vi "AuMT8852B Single-slot Sensitivity Results Query.vi"(8 "error in (no error)":errorcluster, 11 "VISA session":refnum<visa-resource-name>) -> (0 "error out":errorcluster, 2 "error code":i32, 3 "VISA session out":refnum<visa-resource-name>, 4 "Results":T1 {"Overall FER" format="%.2f"; "Current FER" format="%.2f"; "Overall BER" format="%.2f"; "Current BER" format="%.2f"})   [LabVIEW 2017]
doc: "Anritsu MT8852B Bluetooth Tester\n\nReturns the results of the Single-slot Sensitivity test.\n\nOUTPUTS\nResults - measurements made during the test."
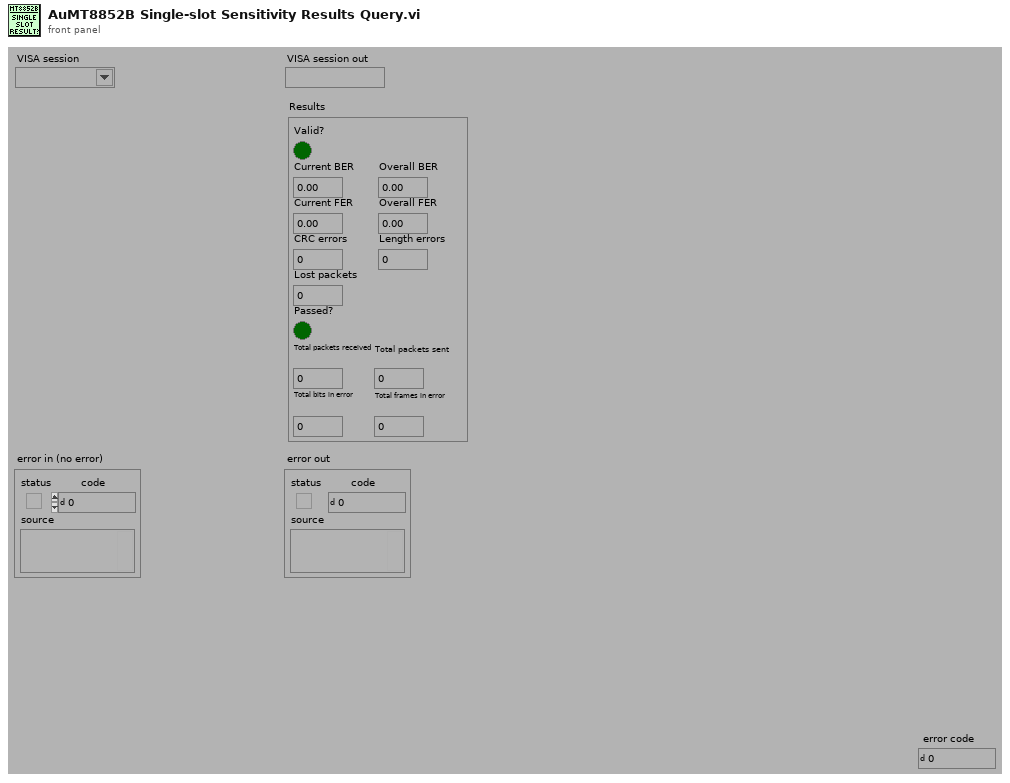
[diagram p1: front panel]
types:
  T1 = cluster{"Valid?":bool, "Current BER":dbl, "Overall BER":dbl, "Current FER":dbl, "Overall FER":dbl, "CRC errors":i32, "Length errors":i32, "Lost packets":i32, "Passed?":bool, "Total packets received":i32, "Total bits in error":i32, "Total frames in error":i32, "Total packets sent":i32}
  T2 = enum16{"Simulate", "Range check", "Cache", "Query instrument status"}
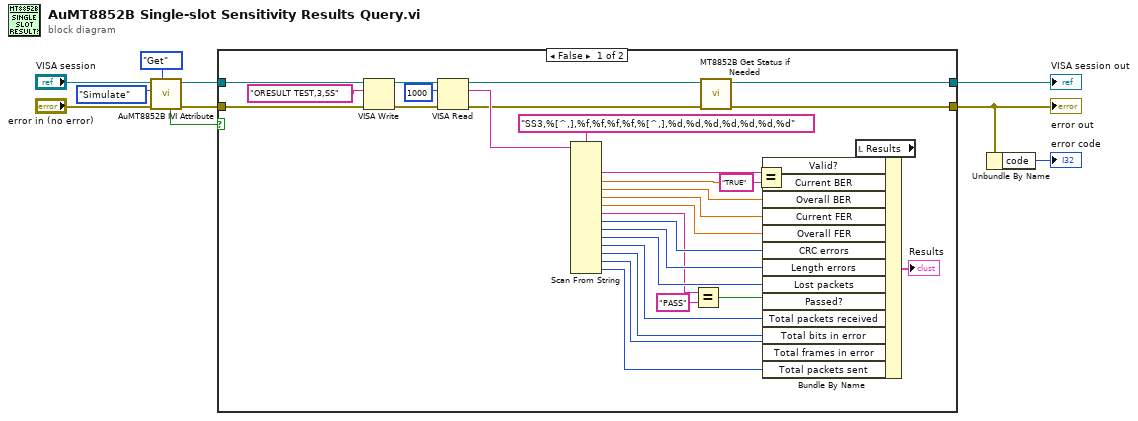
[diagram p0: block diagram]
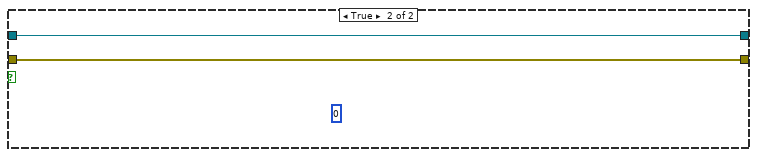
[diagram p2: hidden frame]
diagram:
  n1 = call <instrlib>:"AuMT8852B IVI Attribute.vi"("Set/Get (Set)"=enum16{"Set", "Get"}."Get", "error in (no error)"="error in (no error)", "Flag (Simulate)"=T2."Simulate", "VISA session"="VISA session") -> ("error out"=w7:errorcluster, "VISA session out"=w9:refnum<visa-resource-name>, "Value out"=w3:bool)  [unwired: 5 in]
  n2 = case shown="False" w3 {
    tunnel: [w33 w43] -> w10
    tunnel: [w32 w42] -> w1
    tunnel: w9 -> [w40 w43]
    tunnel: w7 -> [w39 w42]
    frame False {
      n3 = VISA Write(VISA resource name=w40, write buffer="ORESULT TEST,3,SS" ("write buffer (\"\")"), error in (no error)=w39) -> (VISA resource name out=w38:refnum<visa-resource-name>, error out=w37:errorcluster)  [unwired: 1 out]
      n4 = VISA Read(VISA resource name=w38, byte count=u32 1000 ("byte count (0)"), error in (no error)=w37) -> (VISA resource name out=w26:refnum<visa-resource-name>, read buffer=w27:string, error out=w25:errorcluster)  [unwired: 1 out]
      n5 = Scan From String(format string="SS3,%[^,],%f,%f,%f,%f,%[^,],%d,%d,%d,%d,%d,%d,%d" ("Format String"), input string=w27) -> (output 1=w31:string, output 2=w24:dbl, output 3=w23:dbl, output 4=w22:dbl, output 5=w21:dbl, output 6=w15:string, output 7=w18:i32, output 8=w17:i32, output 9=w16:i32, output 10=w14:i32, output 11=w13:i32, output 12=w12:i32, output 13=w11:i32)  [unwired: 15 in, 3 out]
      n6 = Equal?(x=w15, y="PASS") -> (x = y?=w28:bool)
      n7 = call <instrlib>:"MT8852B Get Status if Needed.vi"("error in (no error)"=w25, "VISA session"=w26) -> ("error out"=w32:errorcluster, "VISA session out"=w33:refnum<visa-resource-name>)  [unwired: 8 in]
      n8 = Equal?(x=w31, y="TRUE") -> (x = y?=w30:bool)
      n9 = local read "Results"() -> (w35:T1)
      n10 = Bundle By Name(cluster=w35, "Valid?"=w30, "Current BER"=w24, "Overall BER"=w23, "Current FER"=w22, "Overall FER"=w21, "CRC errors"=w18, "Length errors"=w17, "Lost packets"=w16, "Passed?"=w28, "Total packets received"=w14, "Total bits in error"=w13, "Total frames in error"=w12, "Total packets sent"=w11) -> (→"Results":T1)
    }
    frame True {
      (unwired) u8 0
    }
  }
  "error out" <- w1
  "VISA session out" <- w10
  n11 = Unbundle By Name(w1) -> ("code"=→"error code":i32)
